vi "Offset Widget Actions 2 Transactions.vi"(9 "Number of LBCBs":T5, 11 "Offset Widget Actions":T6) -> (2 "Transactions":T1[](array[typedef]))   [LabVIEW 2013]
uses:
  Global Data/Transactions/Dataset Type.ctl
  Global Data/Transactions/Dataset Source.ctl
  Offset Widget Actions.ctl
  Data Access Objects/Application/Number Of LBCBs.ctl
  Apps/Yes No Button.ctl
  Global Data/Transactions/Dataset Transaction Id.ctl
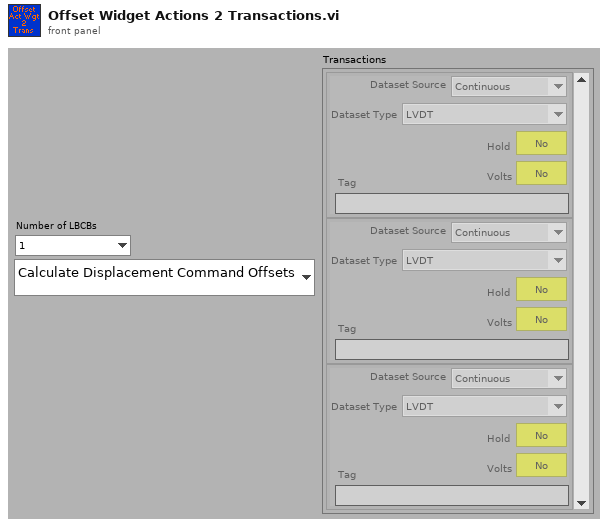
[diagram p1: front panel]
types:
  T1 = typedef "Dataset Transaction Id.ctl" = cluster{"Dataset Source":T2, "Dataset Type":T3, "Hold":T4, "Volts":T4, "Tag":string}
  T2 = typedef "Dataset Source.ctl" = enum16{"Continuous", "Hold", "ED", "Volts", "Offsets"}
  T3 = typedef "Dataset Type.ctl" = enum16{"LVDT", "Load Cell", "Actuator Command", "Servo Error", "Displacement Command", "Displacement", "Force"}
  T4 = typedef "Yes No Button.ctl" = bool
  T5 = typedef "Number Of LBCBs.ctl" = enum16{"1", "2"}
  T6 = typedef "Offset Widget Actions.ctl" = enum16{"Calculate Displacement Command Offsets", "Calculate Displacement Offsets", "Re-Calculate Force Offsets", "Calculate New Force Offsets", "Delete Force Offsets", "Calculate External Sensor Offsets"}
  T7 = typedef "Dataset Source.ctl" = enum16{"LBCB 1", "LBCB 2", "Combined", "External Sensors"}
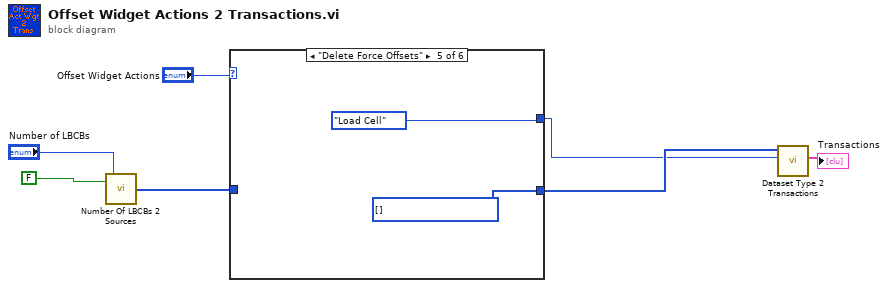
[diagram p0: block diagram]
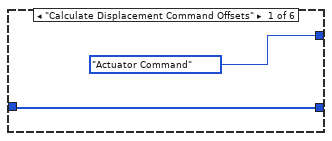
[diagram p2: hidden frame]
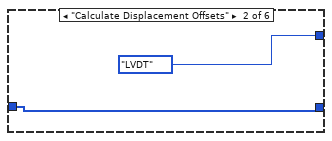
[diagram p3: hidden frame]
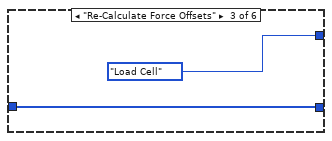
[diagram p4: hidden frame]
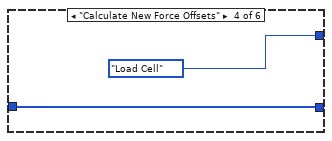
[diagram p5: hidden frame]
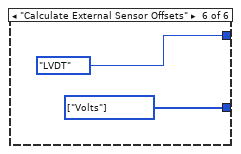
[diagram p6: hidden frame]
diagram:
  n1 = call "Number Of LBCBs 2 Sources.vi"("Number of LBCBs"="Number of LBCBs", "Combined LBCBs"=FALSE) -> ("Sources"=w5:T7[])
  n2 = case shown="\"Delete Force Offsets\"" "Offset Widget Actions" {
    tunnel: [Dataset_Type."Actuator Command" ("Dataset Type") Dataset_Type."LVDT" ("Dataset Type") Dataset_Type."Load Cell" ("Dataset Type") Dataset_Type."Load Cell" ("Dataset Type") Dataset_Type."Load Cell" ("Dataset Type") Dataset_Type."LVDT" ("Dataset Type")] -> w1
    tunnel: w5 -> [w9 w11 w13 w15 _ _]
    tunnel: [w9 w11 w13 w15 w17 w19] -> w4
    frame "Calculate Displacement Command Offsets" {
    }
    frame "Calculate Displacement Offsets" {
    }
    frame "Re-Calculate Force Offsets" {
    }
    frame "Calculate New Force Offsets" {
    }
    frame "Delete Force Offsets" {
      w17 = T2[] [] items=["Continuous", "Hold", "ED", "Volts", "Offsets"] ("Sources")
    }
    frame "Calculate External Sensor Offsets" {
      w19 = T2[] [enum."Volts"] items=["Continuous", "Hold", "ED", "Volts", "Offsets"] ("Sources")
    }
  }
  n3 = call "Dataset Type 2 Transactions.vi"("Dataset Type"=w1, "Sources"=w4) -> ("Transactions"=→"Transactions":T1[])  [unwired: 9 in]
